vi "Read Sync.vi"(8 "error in (no error)":errorcluster, 10 "Number Of Samples":i32, 11 "DeviceRefnum":u64) -> (0 "error out":errorcluster, 1 "Sample Buffer":u8[](array[numeric]), 2 "Samples Read":i32, 3 "DeviceRefnum Out":u64)   [LabVIEW 2014]
doc: "Read a number of samples from the device."
uses:
  <vilib>/Utility/error.llb/Error Cluster From Error Code.vi
  <vilib>/ErrorRing/Error Ring.xnode
panel:
  in  "Sample Buffer In":u8[](array[numeric])
  in  "Samples Read In":i32
  out "function return":i32
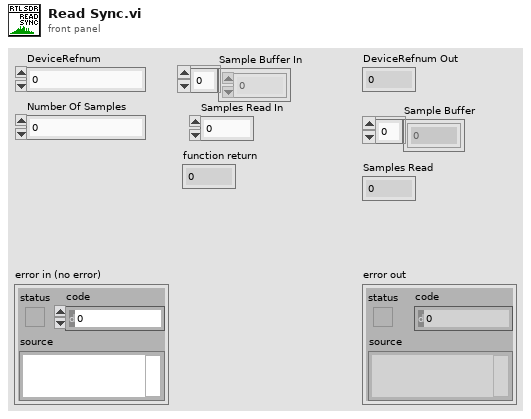
[diagram p1: front panel]
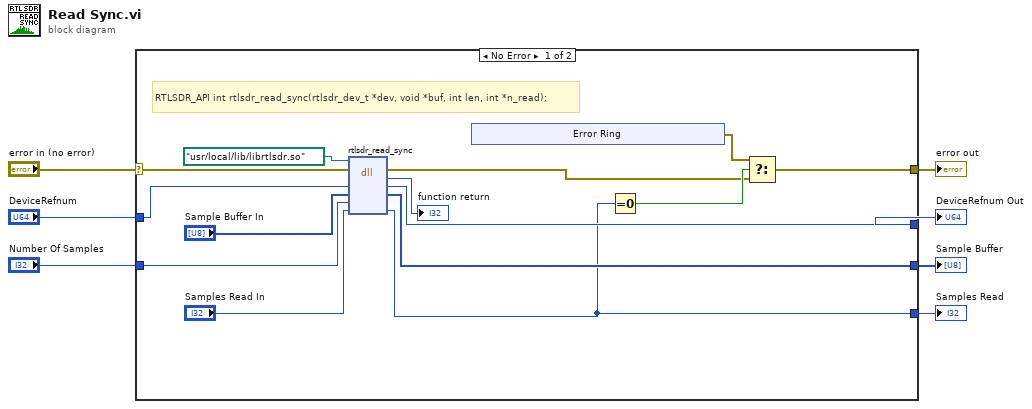
[diagram p0: block diagram]
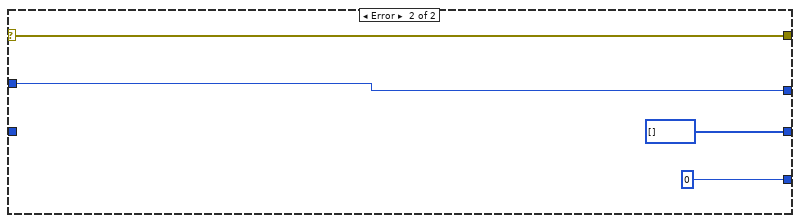
[diagram p2: hidden frame]
diagram:
  n1 = case shown="No Error" "error in (no error)" {
    selector: "error in (no error)" -> [w13 w30]
    tunnel: [w20 u8[] [] ("SampleBuffer")] -> w7
    tunnel: "Number Of Samples" -> [w19 _]
    tunnel: [w12 0 ("SamplesRead")] -> w5
    tunnel: [w9 w30] -> w4
    tunnel: "DeviceRefnum" -> [w17 w28]
    tunnel: [w16 w28] -> w2
    frame No Error {
      # "RTLSDR_API int rtlsdr_read_sync(rtlsdr_dev_t *dev, void *buf, int len, int *n_read);"
      n2 = dll-call lib="C:/Program Files (x86)/National Instruments/LabVIEW 2016/user.lib/rtlsdr/rtlsdr.*" fn="rtlsdr_read_sync"(path in=path "/usr/local/lib/librtlsdr.so", error in=w13, "DeviceRefnum"=w17, "SampleBuffer"="Sample Buffer In", "SamplesToRead"=w19, "SamplesRead"="Samples Read In") -> (error out=w10:errorcluster, "return type"=→"function return":i32, "DeviceRefnum"=w16:u64, "SampleBuffer"=w20:u8[], "SamplesRead"=w12:i32)  [unwired: 2 in, 1 out]
      n3 = xnode "Error Ring"() -> ("error out"=w8:errorcluster)
      n4 = Equal To 0?(x=w12) -> (x = 0?=w11:bool)
      n5 = Select(t=w8, s=w11, f=w10) -> (s? t:f=w9:errorcluster)
    }
    frame Error {
    }
  }
  "Samples Read" <- w5
  "error out" <- w4
  "DeviceRefnum Out" <- w2
  "Sample Buffer" <- w7
